vi "Convert RAW data with DBC.vi"(4 "Signals Map":refnum<vi>, 6 "Frames Map":refnum<vi>, 8 "error in":errorcluster, 9 "XNET Sessions map":refnum<vi>, 10 "ID":u32, 11 "Frame":T1 {"payload" format="%x"; "timestamp" format="%<%.7X\n%x>T"; "type" items=["CAN Data"=0, "CAN Remote"=1, "CAN Bus Error"=2, "CAN 2.0 Data"=8, "CAN FD Data"=16, "CAN FD+BRS Data"=24, "J1939 Data"=192, "Delay"=224, "Log Trigger"=225, "Start Trigger"=226]; "identifier" format="%x"}) -> (0 "error out":errorcluster, 2 "Human Readable DATA":string[][](array[string]))   [LabVIEW 2025, in "CAN-LIN Raw Bus Capture UI.lvlib"]
doc: "This VI finds the signals related to the frames, using DBC. After that converts the RAW CAN Data into Human Readable form."
uses:
  CAN-LIN Raw Bus Capture UI.lvlib
  <vilib>/xnet/xnet.llb/XNET Frame CAN.ctl
  <vilib>/xnet/xnet.llb/XNET Frame Type CAN.ctl
  <vilib>/xnet/xnet.llb/XNET Convert (Frame CAN to Signal).vi
  <resource>/objmgr/xnet.rc
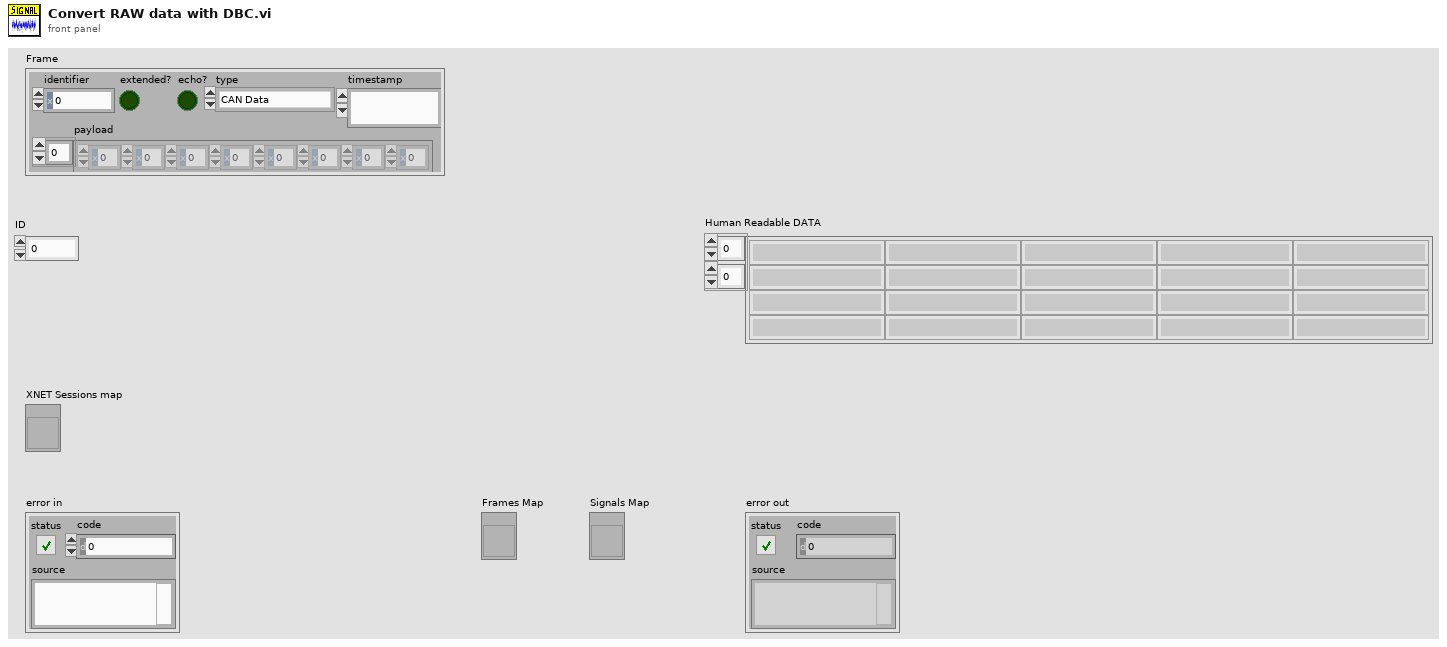
[diagram p1: front panel]
types:
  T1 = typedef "XNET Frame CAN.ctl" = cluster{"timestamp":timestamp, "payload":u8[], "identifier":u32, "type":T2, "extended?":bool, "echo?":bool}
  T2 = typedef "XNET Frame Type CAN.ctl" = u8
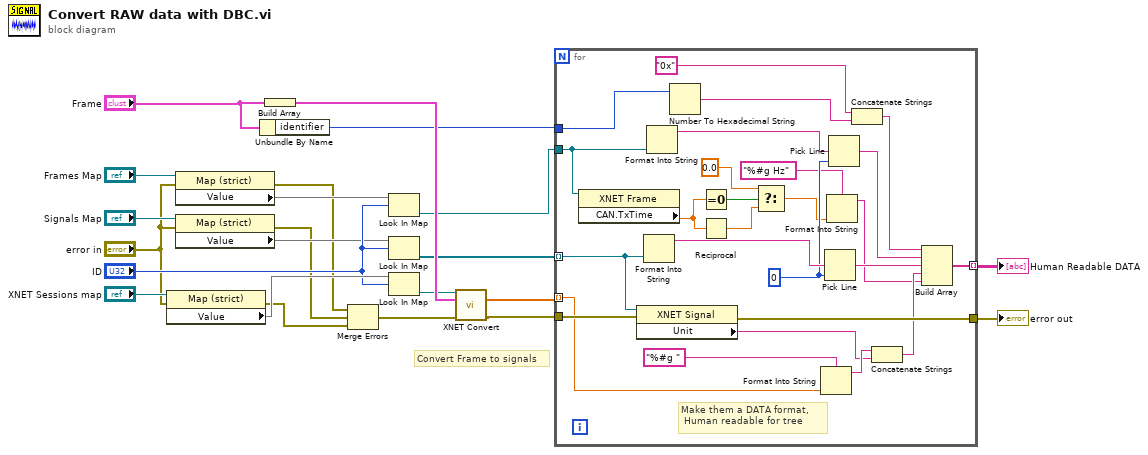
[diagram p0: block diagram]
diagram:
  # "Convert Frame to signals"
  n1 = property class="Map (strict)"(reference="XNET Sessions map", error in="error in") -> (error out=w2:errorcluster, "Value"=w12:map{u32, refnum<k21>})  [unwired: 1 out]
  n2 = property class="Map (strict)"(reference="Frames Map", error in="error in") -> (error out=w4:errorcluster, "Value"=w8:map{u32, refnum<k21>})  [unwired: 1 out]
  n3 = property class="Map (strict)"(reference="Signals Map", error in="error in") -> (error out=w3:errorcluster, "Value"=w5:map{u32, refnum<k21>[]})  [unwired: 1 out]
  n4 = Unbundle By Name("Frame") -> ("identifier"=w17:u32)
  n5 = Build Array("Frame") -> (w19:T1[])
  n6 = Merge Errors(w4, w3, w2) -> (w1:errorcluster)
  n7 = Look In Map(map=w8, key="ID") -> (value=w15:refnum<k21>)  [unwired: 1 in, 1 out]
  n8 = Look In Map(map=w5, key="ID") -> (value=w14:refnum<k21>[])  [unwired: 1 in, 1 out]
  n9 = Look In Map(map=w12, key="ID") -> (value=w10:refnum<k21>)  [unwired: 1 in, 1 out]
  n10 = call-poly <vilib>:"XNET Convert.vi"("session in"=w10, "frame data"=w19, "error in (no error)"=w1) -> ("signal data"=w20:dbl[], "error out"=w16:errorcluster)  [unwired: 11 out]
  n11 = for {
    tunnel: w20 -> [w23] mode=indexing
    tunnel: w14 -> [w34] mode=indexing
    tunnel: [w48] -> w22 mode=indexing
    tunnel: w15 -> [w31]
    tunnel: w17 -> [w42]
    tunnel: [w33] -> w21
    tunnel: w16 -> [w35]
    w44 = 0 ("line index")
    # "Make them a DATA format,\n Human readable for tree"
    n12 = property class="XNET Frame"(reference=w31) -> ("CAN.TxTime"=w27:dbl)  [unwired: 1 in, 2 out]
    n13 = property class="XNET Signal"(reference=w34, error in=w35) -> (error out=w33:errorcluster, "Unit"=w36:string)  [unwired: 1 out]
    n14 = Format Into String(w34) -> (resulting string=w47:string)  [unwired: 3 in, 1 out]
    n15 = Format Into String(w31) -> (resulting string=w45:string)  [unwired: 3 in, 1 out]
    n16 = Number To Hexadecimal String(2:w42) -> (0:w40:string)  [unwired: 1 in]
    n17 = Equal To 0?(x=w27) -> (x = 0?=w30:bool)
    n18 = Reciprocal(x=w27) -> (1/x=w26:dbl)
    n19 = Select(t=0.0, s=w30, f=w26) -> (s? t:f=w29:dbl)
    n20 = Format Into String(format string="%#g ", w23) -> (resulting string=w38:string)  [unwired: 2 in, 1 out]
    n21 = Pick Line(multi-line string=w47, line index=w44) -> (output string=w46:string)  [unwired: 1 in]
    n22 = Format Into String(format string="%#g Hz", w29) -> (resulting string=w24:string)  [unwired: 2 in, 1 out]
    n23 = Pick Line(multi-line string=w45, line index=w44) -> (output string=w43:string)  [unwired: 1 in]
    n24 = Concatenate Strings("0x" ("string"), w40) -> (w39:string)
    n25 = Concatenate Strings(w38, w36) -> (w32:string)
    n26 = Build Array(w39, w43, w46, w32, w24) -> (w48:string[])
  }
  "Human Readable DATA" <- w22
  "error out" <- w21
